vi "update.vi"(8 "error in":errorcluster, 10 "settings cluster":T3, 11 "FPGA VI ref":T2) -> (0 "error out":errorcluster)   [LabVIEW 2010]
uses:
  type definitions/settings_cluster.ctl
  common_typedefs/channels_cluster.ctl
  type definitions/gate_cluster.ctl
  common_typedefs/gate_parameters_cluster.ctl
  FPGA_VI_reference.ctl
  <vilib>/rvi/interface/nirviReadWriteControl/nirviReadWriteControl.xnode
  <vilib>/rvi/interface/common/niFpgaNodeNameForErrorReporting.ctl
  <vilib>/rvi/errors/niLvFpgaWhatHappensToTopLevelVI.ctl
  <vilib>/Utility/error.llb/Error Cluster From Error Code.vi
  <vilib>/rvi/errors/niLvFpgaAdjustHostInterfaceError.vi
  NiFpgaLv.dll
panel:
  out "pixel values cluster":T1
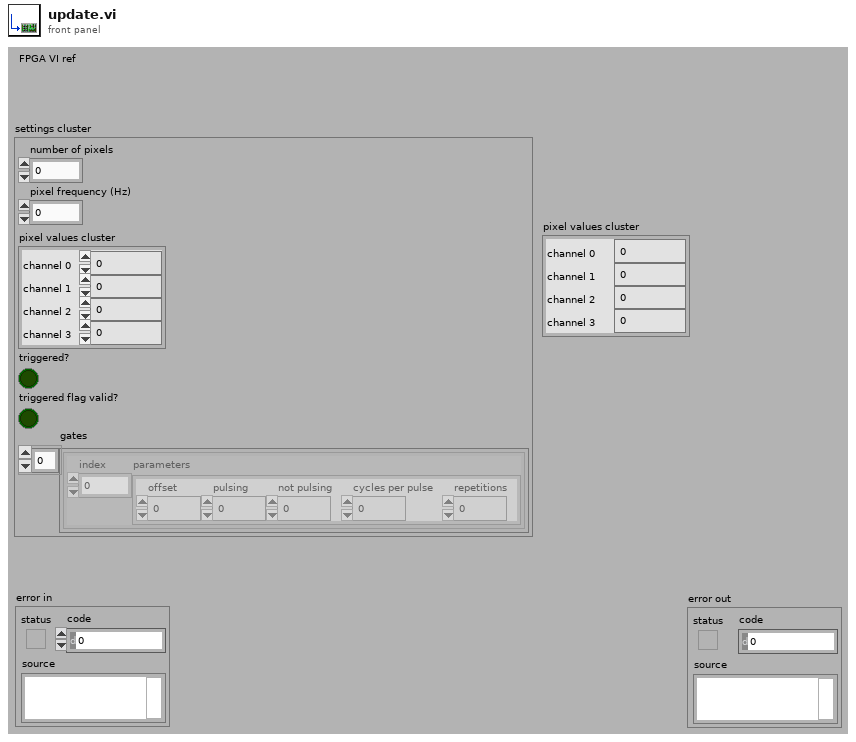
[diagram p1: front panel]
types:
  T1 = typedef "channels_cluster.ctl" = cluster{"channel 0":u32, "channel 1":u32, "channel 2":u32, "channel 3":u32}
  T2 = typedef "FPGA_VI_reference.ctl" = refnum<k20>
  T3 = typedef "settings_cluster.ctl" = cluster{"number of pixels":i64, "pixel frequency (Hz)":dbl, "pixel values cluster":T1, "triggered?":bool, "triggered flag valid?":bool, "gates":T4[]}
  T4 = typedef "gate_cluster.ctl" = cluster{"index":i32, "parameters":T5}
  T5 = typedef "gate_parameters_cluster.ctl" = cluster{"offset":i64, "pulsing":i64, "not pulsing":i64, "cycles per pulse":i64, "repetitions":i64}
  T6 = typedef "niFpgaNodeNameForErrorReporting.ctl" = enum16{"Open FPGA VI Reference", "Read/Write Control", "Invoke Method: Abort", "Invoke Method: Acknowledge IRQ", "Invoke Method: Download", "Invoke Method: FIFO.Configure", "Invoke Method: FIFO.Read", "Invoke Method: FIFO.Start", "Invoke Method: FIFO.Stop", "Invoke Method: FIFO.Write", "Invoke Method: Reset", "Invoke Method: Run", "Invoke Method: Wait on IRQ", "Close FPGA VI Reference"}
  T7 = typedef "niLvFpgaWhatHappensToTopLevelVI.ctl" = enum16{"top level VI scripted behind XNode", "top level VI inlined behind XNode"}
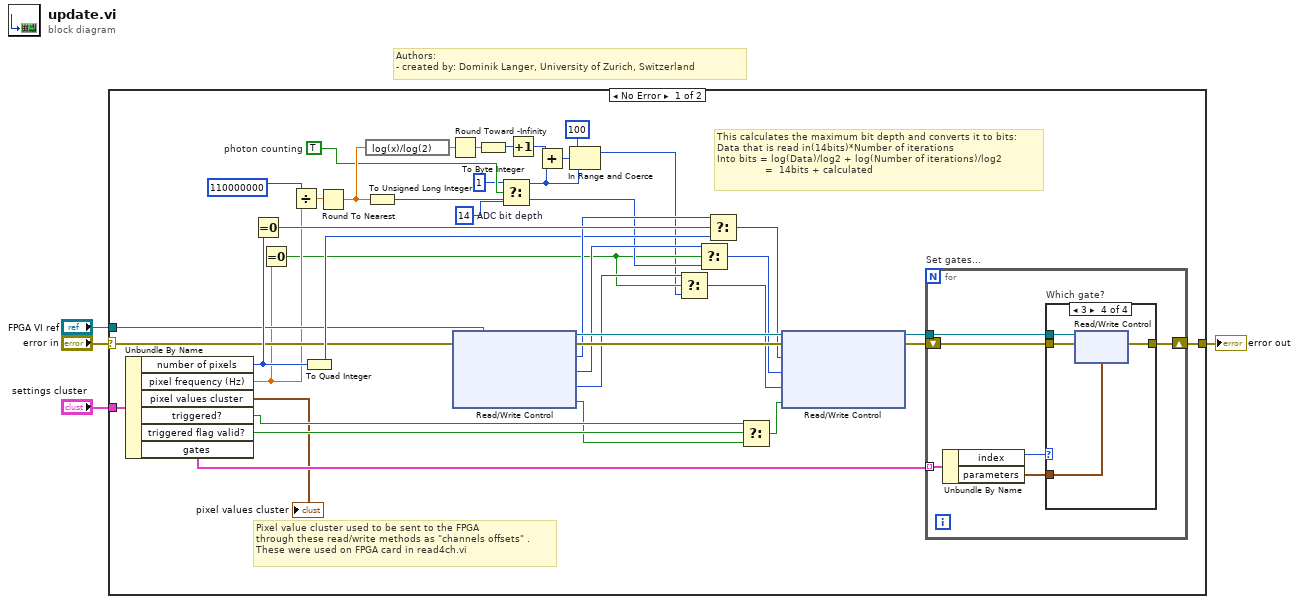
[diagram p0: block diagram]
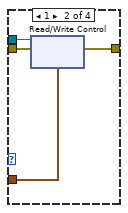
[diagram p3: hidden frame]
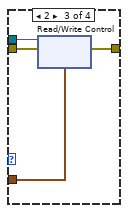
[diagram p4: hidden frame]
diagram:
  # "Authors: \n- created by: Dominik Langer, University of Zurich, Switzerland"
  n1 = case shown="No Error" "error in" {
    selector: "error in" -> [w30 w425]
    tunnel: "settings cluster" -> [w31 _]
    tunnel: [w25 w425] -> w2
    tunnel: "FPGA VI ref" -> [w29 _]
    frame No Error {
      w8 = TRUE  # photon counting
      w7 = i8 14  # ADC bit depth
      # "Pixel value cluster used to be sent to the FPGA\nthrough these read/write methods as \"channels offsets\" .\nThese were used on FPGA card in read4ch.vi"
      # "This calculates the maximum bit depth and converts it to bits:\nData that is read in(14bits)*Number of iterations\nInto bits = log(Data)/log2 + log(Number of iterations)/log2\n                =  14bits + calculated"
      n2 = Unbundle By Name(w31) -> ("number of pixels"=w42:i64, "pixel frequency (Hz)"=w22:dbl, "pixel values cluster"=→"pixel values cluster":T1, "triggered?"=w33:bool, "triggered flag valid?"=w34:bool, "gates"=w27:T4[])
      n3 = Equal To 0?(x=w42) -> (x = 0?=w41:bool)
      n4 = Equal To 0?(x=w22) -> (x = 0?=w19:bool)
      n5 = Divide(x=110000000, y=w22) -> (x/y=w21:dbl)
      n6 = To Quad Integer(1:w42) -> (0:w39:i64)
      n7 = Round To Nearest(number=w21) -> (nearest integer value=w12:dbl)
      n8 = expression code="log(x)/log(2)"(w12) -> (w13:dbl)
      n9 = To Unsigned Long Integer(number=w12) -> (unsigned 32bit integer=w20:u32)
      n10 = Round Toward -Infinity(1:w13) -> (0:w14:dbl)
      n11 = xnode "Read/Write Control"("FPGA VI Reference In"=w29, "error in"=w30) -> ("FPGA VI Reference Out"=w44:T2, "error out"=w43:errorcluster, "number of pixels"=w40:i64, "iterations per pixel"=w37:u32, "maximum bit depth"=w35:i8, "wait for trigger?"=w28:bool)
      n12 = To Byte Integer(number=w14) -> (8bit integer=w15:i8)
      n13 = Select(t=i8 1, s=w8, f=w7) -> (s? t:f=w9:i8)
      n14 = Increment(x=w15) -> (x+1=w16:i8)
      n15 = Add(x=w16, y=w9) -> (x+y=w17:i8)
      n16 = In Range and Coerce(upper limit=i8 100, x=w17, lower limit=w9) -> (coerced(x)=w11:i8)  [unwired: 1 out]
      n17 = Select(t=w35, s=w19, f=w11) -> (s? t:f=w10:i8)
      n18 = Select(t=w37, s=w19, f=w20) -> (s? t:f=w36:u32)
      n19 = Select(t=w40, s=w41, f=w39) -> (s? t:f=w38:i64)
      n20 = Select(t=w33, s=w34, f=w28) -> (s? t:f=w32:bool)
      n21 = xnode "Read/Write Control"("FPGA VI Reference In"=w44, "error in"=w43, "number of pixels"=w38, "iterations per pixel"=w36, "maximum bit depth"=w10, "wait for trigger?"=w32) -> ("FPGA VI Reference Out"=w24:T2, "error out"=w26:errorcluster)
      n22 = for "Set gates..." {
        tunnel: w27 -> [w50] mode=indexing
        shift-right: [w46] -> w25
        shift-left: w26 -> [w49]
        tunnel: w24 -> [w48]
        n23 = Unbundle By Name(w50) -> ("index"=w47:i32, "parameters"=w45:T5)
        n24 = case "Which gate?" shown="3" w47 {
          tunnel: w49 -> [w51 w55 w101 w149]
          tunnel: w48 -> [_ w54 w103 w150]
          tunnel: [w51 w53 w100 w148] -> w46
          tunnel: w45 -> [_ w52 w102 w151]
          frame Default {
          }
          frame 1 {
            n25 = xnode "Read/Write Control"("FPGA VI Reference In"=w54, "error in"=w55, "gate 1"=w52) -> ("error out"=w53:errorcluster)  [unwired: 1 out]
          }
          frame 2 {
            n26 = xnode "Read/Write Control"("FPGA VI Reference In"=w103, "error in"=w101, "gate 2"=w102) -> ("error out"=w100:errorcluster)  [unwired: 1 out]
          }
          frame 3 {
            n27 = xnode "Read/Write Control"("FPGA VI Reference In"=w150, "error in"=w149, "gate 3"=w151) -> ("error out"=w148:errorcluster)  [unwired: 1 out]
          }
        }
      }
    }
    frame Error {
    }
  }
  "error out" <- w2
